vi "DriverStation Are Outputs Enabled.vi"(8 "error in":errorcluster) -> (0 "error out":errorcluster, 3 "OutputsEnabled?":bool)   [LabVIEW 2026, in "MrcLib.lvlib"]
doc: "Are actuators and output I/O enabled. Outputs will be disabled due to loss of communications, overvoltage or brownout conditions on the input power to the robot controller."
uses:
  MrcLib.lvlib
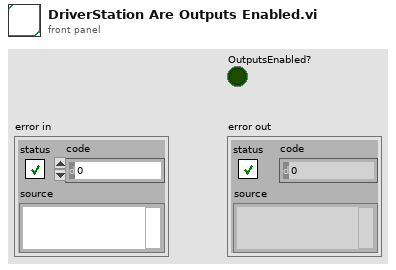
[diagram p1: front panel]
types:
  T1 = typedef "MrcLib.lvlib/MRC_ControlData.ctl" = cluster{"controlFlags":u32, "matchTime":u16, "currentOpMode":u64, "gameDataLength":u8, "gameData":cluster{"gameData 0":u8, "gameData 1":u8, "gameData 2":u8, "gameData 3":u8, "gameData 4":u8, "gameData 5":u8, "gameData 6":u8, "gameData 7":u8}}
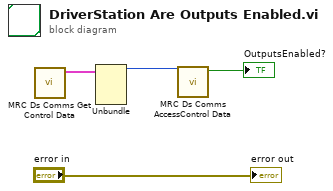
[diagram p0: block diagram]
diagram:
  n1 = call "MRC Ds Comms Get Control Data.vi"() -> ("data out"=w3:T1)  [unwired: 10 in, 1 out]
  n2 = Unbundle(w3) -> ("controlFlags"=w2:u32)  [unwired: 4 out]
  n3 = call "MRC Ds Comms AccessControl Data.vi"("controlFlag"=w2) -> ("Enabled"=→"OutputsEnabled?":bool)  [unwired: 7 in, 3 out]
  "error out" <- "error in"
